vi "Update Component Map from Array.vi"(10 "Array of components in":T2(array[cluster]), 11 "Game Board Components[] in":T1(c390)) -> (3 "Game Board Components[] out":T1(c390))   [LabVIEW 2024, in "Game Board.lvclass"]
doc: "MIT Licence\nCopyright (c) 2024 David Grollier"
uses:
  Game Board.lvclass
  Game Board Component/Game Board Component.lvclass
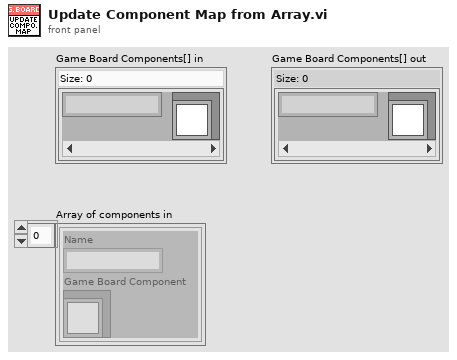
[diagram p1: front panel]
types:
  T1 = map{string, refnum<class "Game Board Component.lvclass">}
  T2 = cluster{"Name":string, "Game Board Component":refnum<class "Game Board Component.lvclass">}[]
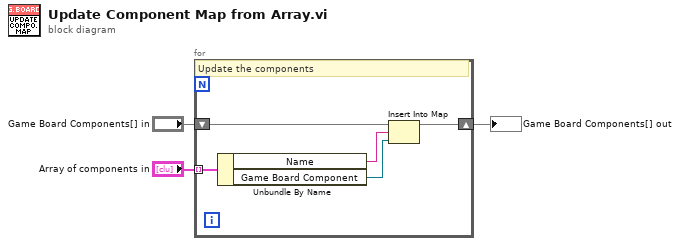
[diagram p0: block diagram]
diagram:
  n1 = for {
    shift-right: [w7] -> w3
    shift-left: "Game Board Components[] in" -> [w8]
    tunnel: "Array of components in" -> [w6] mode=indexing
    # "Update the components"
    n2 = Unbundle By Name(w6) -> ("Name"=w5:string, "Game Board Component"=w4:refnum<class "Game Board Component.lvclass">)
    n3 = Insert Into Map(map in=w8, key=w5, value=w4) -> (map out=w7:T1)  [unwired: 2 out]
  }
  "Game Board Components[] out" <- w3
